vi "Launch App.vi"() -> ()   [LabVIEW 2019]
doc: "Developed by Kevin Thompson\nkevin@thompsonengineering.net\n\nCopyright 2018-2020\nThompson Engineering, LLC"
uses:
  Source/Common/DataTypes/TD GetSet ActionSelect--enum.ctl
  Source/Common/Startup/TD LaunchData--cluster.ctl
  Source/Common/Startup/TD LaunchState--enum.ctl
  Source/Common/Startup/GBL System.vi
  Source/Common/ErrorHandler/ErrorHandler.lvclass
panel:
  out "FP Msg":string="Launching AVC 2.0\nPlease Wait . . ."
  in  "MinimizeLauncher":bool
  out "StatusStr.Launcher":string
  in  "AbortSystemStart":bool
  out "AppVer":string="Ichor Systems AVC2 - Development Mode" caption="Version:"
  # "Launching AVC 2.0\nPlease Wait . . ."
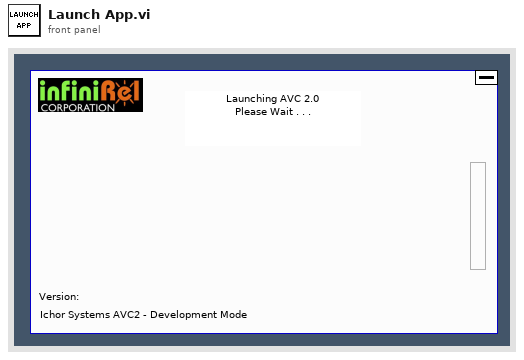
[diagram p1: front panel]
types:
  T1 = typedef "TD GetSet ActionSelect--enum.ctl" = enum16{"Init", "Get", "Set"}
  T2 = enum32{"Invalid", "Default", "Floating", "Floating/Auto-Hide", "Modal"}
  T3 = enum32{"invalid app kind", "Development System", "Run Time System", "Student Edition", "Embedded LabVIEW", "Evaluation", "Custom"}
  T4 = enum32{"Invalid", "Standard", "Closed", "Hidden", "Minimized", "Maximized"}
  T5 = typedef "TD LaunchState--enum.ctl" = enum16{"Started", "Stopped"}
  T6 = typedef "TD LaunchData--cluster.ctl" = cluster{"Time Stamp":timestamp, "LaunchState":T5, "Error":errorcluster}
  T7 = typedef "TD Pathnames--cluster.ctl" = cluster{"RunTimeSys?":bool, "AppFolder":path, "ExecutablePath":path, "ConfigFolder":path, "DataLogFolder":path, "SystemLogFolder":path, "SeqFolder":path, "MainStartupPathname":path, "MainUIPathname":path, "SystemEventsFile":path, "SeqEventsFile":path, "Config SettingsFile":path, "DAQ IOConfigFile":path, "SystemSimulation":bool}
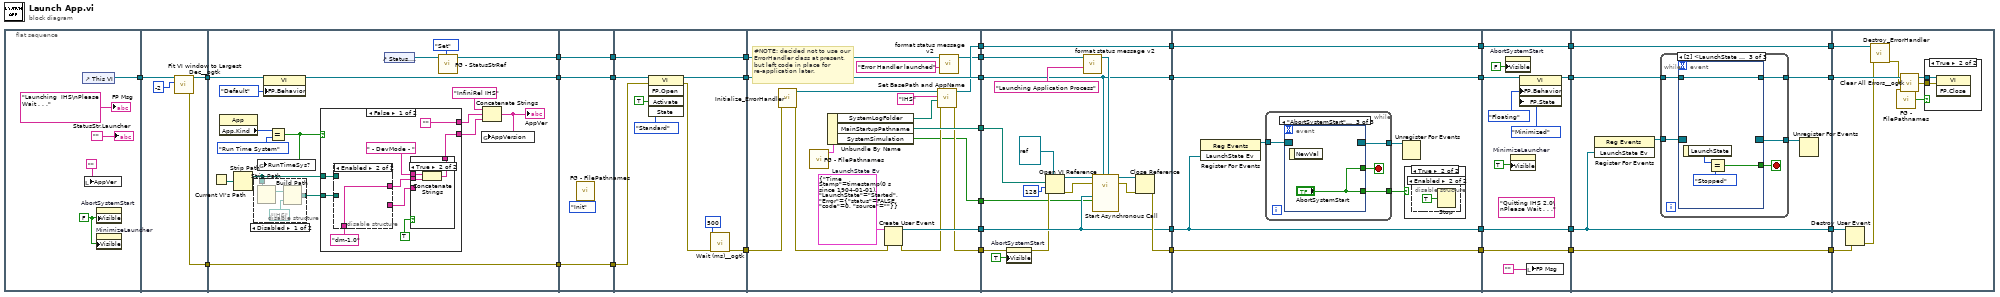
[diagram p0: block diagram]
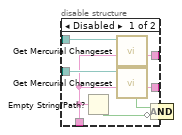
[diagram p3: hidden frame]
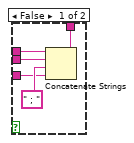
[diagram p4: hidden frame]
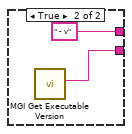
[diagram p5: hidden frame]
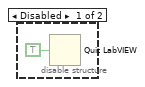
[diagram p7: hidden frame]
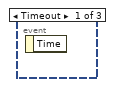
[diagram p8: hidden frame]
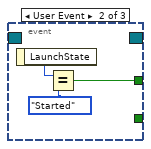
[diagram p9: hidden frame]
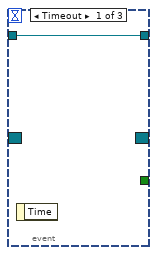
[diagram p10: hidden frame]
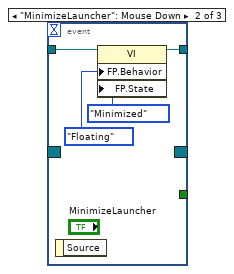
[diagram p11: hidden frame]
diagram:
  n1 = flat-sequence {
    tunnel: [w40] -> w12
    tunnel: [w42] -> w35
    tunnel: [w41] -> w34
    tunnel: w12 -> [w43]
    tunnel: w35 -> [w53]
    tunnel: w34 -> [w56]
    tunnel: [w56] -> w32
    tunnel: [w52] -> w30
    tunnel: [w48] -> w1
    tunnel: w32 -> [w96]
    tunnel: [w96] -> w31
    tunnel: w30 -> [w95]
    tunnel: [w95] -> w29
    tunnel: [w94] -> w3
    tunnel: w1 -> [w94]
    tunnel: w31 -> [w102]
    tunnel: w29 -> [w103]
    tunnel: [w99] -> w33
    tunnel: [w101] -> w25
    tunnel: w3 -> [w97]
    tunnel: [w97] -> w2
    tunnel: w33 -> [w119]
    tunnel: [w112] -> w28
    tunnel: [w122] -> w27
    tunnel: [w121] -> w26
    tunnel: w25 -> [w121]
    tunnel: [w114] -> w11
    tunnel: [w110] -> w9
    tunnel: [w109] -> w5
    tunnel: [w108] -> w4
    tunnel: w2 -> [w107]
    tunnel: w28 -> [w132]
    tunnel: w27 -> [w134]
    tunnel: w26 -> [w124]
    tunnel: [w135] -> w24
    tunnel: [w134] -> w23
    tunnel: [w124] -> w19
    tunnel: w11 -> [w130]
    tunnel: [w129] -> w10
    tunnel: w9 -> [w129]
    tunnel: w5 -> [w128]
    tunnel: w4 -> [w127]
    tunnel: w24 -> [w147]
    tunnel: w23 -> [w144]
    tunnel: [w147] -> w22
    tunnel: [w144] -> w21
    tunnel: [w142] -> w20
    tunnel: w19 -> [w142]
    tunnel: w10 -> [w141]
    tunnel: [w141] -> w7
    tunnel: w22 -> [w167]
    tunnel: w21 -> [w166]
    tunnel: w20 -> [w164]
    tunnel: [w167] -> w18
    tunnel: [w166] -> w17
    tunnel: [w163] -> w16
    tunnel: [w160] -> w8
    tunnel: w7 -> [w160]
    tunnel: w18 -> [w174]
    tunnel: w17 -> [w172]
    tunnel: w16 -> [w169]
    tunnel: [w174] -> w15
    tunnel: [w168] -> w14
    tunnel: [w172] -> w13
    tunnel: w8 -> [w170]
    tunnel: [w170] -> w6
    tunnel: w15 -> [w195]
    tunnel: w14 -> [w194]
    tunnel: w13 -> [w196]
    tunnel: w6 -> [w193]
    frame #0 {
      w38 = FALSE ("Visible")
      n2 = control-ref of="This VI"() -> (w40:refnum<vi>)
      n3 = local write "AppVer"("") -> ()
      n4 = property on="MinimizeLauncher" class="Bool"("Visible"=w38) -> ()  [unwired: 2 in, 2 out]
      n5 = property on="AbortSystemStart" class="Bool"("Visible"=w38) -> ()  [unwired: 2 in, 2 out]
      "StatusStr.Launcher" <- ""
      "FP Msg" <- "Launching  IHS\nPlease Wait . . ." ("FP Msg")
    }
    frame #1 {
      n6 = call <userlib>:"Fit VI window to Largest Dec__ogtk.vi"("border spacing (2 px)"=-2, "VI Ref (calling VI)"=w43) -> ("error out"=w41:errorcluster, "dup VI Ref"=w42:refnum<vi>)  [unwired: 4 in]
    }
    frame #2 {
      n7 = Current VI's Path() -> (path=w47:path)
      n8 = property class="App"() -> ("App.Kind"=w61:T3)  [unwired: 2 in, 2 out]
      n9 = Strip Path(path=w47) -> (stripped path=w46:path)  [unwired: 1 out]
      n10 = disable-structure shown="Disabled" {
        disable-tunnel: w46 -> [w65 _]
        disable-tunnel: [w62 _] -> w45
        frame Disabled {
          n11 = Strip Path(path=w65) -> (stripped path=w64:path)  [unwired: 1 out]
          n12 = Build Path(base path=w64, name or relative path=path "IHS") -> (appended path=w62:path)
        }
        frame Enabled {
        }
      }
      n13 = property class="VI"(reference=w53, "FP.Behavior"=T2."Default" ("Front Panel Window:Behavior")) -> (reference out=w52:refnum<vi>)  [unwired: 1 in, 1 out]
      n14 = Equal?(x=w61, y=T3."Run Time System" ("Application:Kind")) -> (x = y?=w57:bool)
      n15 = global write "GBL System.vi" "RunTimeSys?"(w57) -> ()
      n16 = case shown="False" w57 {
        tunnel: [w70 w92] -> w59
        tunnel: ["" " - v" ("string")] -> w60
        tunnel: w46 -> [w73 _]
        tunnel: w45 -> [w69 _]
        frame False {
          n17 = disable-structure shown="Enabled" {
            disable-tunnel: w73 -> [w81 _]
            disable-tunnel: [w80 w82] -> w71
            disable-tunnel: w69 -> [w79 _]
            disable-tunnel: [w75 _] -> w68
            disable-tunnel: "dm-1.0" -> [w76 w82]
            frame Disabled {
              n18 = Empty String/Path?(string/path=w76) -> (empty?=w77:bool)
              n19 = call "Get Mercurial Changeset.vi"("not found string (\"\")"=w76, "Path"=w81) -> ("Change Set String"=w80:string)  [unwired: 6 in, 3 out]
              n20 = call "Get Mercurial Changeset.vi"("not found string (\"\")"=w76, "Path"=w79) -> ("Change Set String"=w75:string, "repo error?"=w78:bool)  [unwired: 6 in, 2 out]
              n21 = Compound Arithmetic op=AND(w78, invert w77) -> ()  [unwired: 1 out]
            }
            frame Enabled {
            }
          }
          n22 = case shown="True" TRUE {
            tunnel: " - DevMode - " -> [w87 w90]
            tunnel: w71 -> [w86 w88]
            tunnel: [w85 w89] -> w70
            tunnel: w68 -> [w83 _]
            frame False {
              n23 = Concatenate Strings(w87, w86, " ; ", w83) -> (w85:string)
            }
            frame True {
              n24 = Concatenate Strings(w90, w88) -> (w89:string)
            }
          }
        }
        frame True {
          n25 = call <userlib>:"MGI Get Executable Version.vi"() -> ("Version"=w92:string)  [unwired: 7 in]
        }
      }
      n26 = control-ref of="Status.Launcher"() -> (w50:refnum<vi>)
      n27 = call "FG - StatusStrRef.vi"("StatusStr Ref in"=w50, "action (Get)"=TD_GetSet_ActionSelect--enum."Set") -> ("StatusStr Ref out"=w48:refnum<vi>)  [unwired: 7 in, 1 out]
      n28 = Concatenate Strings("InfiniRel IHS" ("string"), w60, w59) -> (w55:string)
      "AppVer" <- w55
      n29 = global write "GBL System.vi" "AppVersion"(w55) -> ()
    }
    frame #3 {
      n30 = call "FG - FilePathnames.vi"("action (Get)"=TD_GetSet_ActionSelect--enum."Init") -> ()  [unwired: 3 in, 2 out]
    }
    frame #4 {
      n31 = invoke class="VI" method="FP.Open"(reference=w103, error in=w102, "Activate"=TRUE ("Activate?"), "State"=T4."Standard") -> (reference out=w101:refnum<vi>, error out=w100:errorcluster)  [unwired: 1 in, 3 out]
      n32 = call <userlib>:"Wait (ms)__ogtk.vi"("error in (no error)"=w100, "milliseconds to wait"=u32 500) -> ("error out"=w99:errorcluster)  [unwired: 8 in, 1 out]
    }
    frame #5 {
      w120 = T6 {"Time Stamp"=timestamp(0 s since 1904-01-01), "LaunchState"=enum."Started", "Error"={"status"=FALSE, "code"=0, "source"=""}}  # LaunchState Ev
      # "#NOTE: decided not to use our\nErrorHandler class at present,\nbut left code in place for\nre-application later."
      n33 = call "Initialize_ErrorHandler.vi"("error in (no error)"=w119) -> ("error out"=w118:errorcluster, "ErrorHandler out"=w117:refnum<class "ErrorHandler.lvclass">)  [unwired: 9 in]
      n34 = call "FG - FilePathnames.vi"() -> ("FilePaths out"=w116:T7)  [unwired: 4 in, 1 out]
      n35 = Unbundle By Name(w116) -> ("SystemLogFolder"=w115:path, "MainStartupPathname"=w114:path, "SystemSimulation"=w109:bool)
      n36 = Create User Event(user event datatype=w120, error in=w118) -> (user event=w122:refnum<user-event>, error out=w113:errorcluster)
      n37 = call "Set BasePath and AppName.vi"("error in (no error)"=w113, "ErrorLogBasePath"=w115, "AppName"="IHS", "ErrorHandler in"=w117) -> ("error out"=w112:errorcluster, "ErrorHandler out"=w110:refnum<class "ErrorHandler.lvclass">)  [unwired: 6 in]
      n38 = call <vilib>:"format status message v2.vi"("status msg"="Error Handler launched", "Str Refnum"=w107) -> ("Str Refnum out"=w108:refnum<vi>)  [unwired: 5 in, 4 out]
    }
    frame #6 {
      n39 = property on="AbortSystemStart" class="Bool"(error in=w132, "Visible"=TRUE) -> (error out=w131:errorcluster)  [unwired: 1 in, 1 out]
      n40 = Open VI Reference(type specifier VI Refnum (for type only)=refnum<vi> refnum, vi path=w130, options=128, error in (no error)=w131) -> (vi reference=w139:refnum<vi>, error out=w136:errorcluster)  [unwired: 2 in]
      n41 = call <vilib>:"format status message v2.vi"("status msg"="Launching Application Process", "Str Refnum"=w127) -> ("Str Refnum out"=w125:refnum<vi>)  [unwired: 5 in, 4 out]
      n42 = call-by-ref "Start Asynchronous Call"(reference=w139, error in=w136, "Splash StatusRef"=w125, "Splash VI Ref"=w124, "Simulation?"=w128, "LaunchState Ev"=w134) -> (reference out=w138:refnum<vi>, error out=w137:errorcluster)  [unwired: 8 in]
      n43 = Close Reference(reference=w138, error in (no error)=w137) -> (error out=w135:errorcluster)
    }
    frame #7 {
      n44 = register-events(w144) -> (reference out=w146:refnum<event-registration>)  [unwired: 2 in, 1 out]
      n45 = while {
        tunnel: w146 -> [w153]
        tunnel: [w152] -> w145
        tunnel: [w150] -> w143
        stop <- w151 stop-if-true
        n46 = event shown="[2] \"AbortSystemStart\": Value Change" {
          selector: w153 -> [_ _ _]
          dyn-events: [_ _ _] -> w152
          timeout: _ -> [_ _ _]
          tunnel: [_ w154 "AbortSystemStart"] -> w151
          tunnel: [_ _ "AbortSystemStart"] -> w150
          event Timeout {
            n47 = event-data() -> ()  [unwired: 1 in, 1 out]
          }
          event User Event {
            n48 = event-data() -> ("LaunchState"=w156:T5)  [unwired: 1 in]
            n49 = Equal?(x=w156, y=TD_LaunchState--enum."Started") -> (x = y?=w154:bool)
          }
          event "AbortSystemStart": Value Change {
            n50 = event-data() -> ()  [unwired: 1 in, 1 out]
          }
        }
      }
      n51 = Unregister For Events(event registration refnum=w145) -> ()  [unwired: 1 in, 1 out]
      n52 = case shown="True" w143 {
        frame False {
        }
        frame True {
          n53 = disable-structure shown="Enabled" {
            frame Disabled {
              n54 = Quit LabVIEW(quit? (T)=TRUE) -> ()
            }
            frame Enabled {
              n55 = Stop(stop? (T)=TRUE) -> ()
            }
          }
        }
      }
    }
    frame #8 {
      (unwired) "Quitting IHS 2.0\nPlease Wait . . ." ("FP Msg")
      n56 = property on="AbortSystemStart" class="Bool"("Visible"=FALSE) -> ()  [unwired: 2 in, 2 out]
      n57 = property on="MinimizeLauncher" class="Bool"("Visible"=TRUE) -> ()  [unwired: 2 in, 2 out]
      n58 = property class="VI"(reference=w164, "FP.Behavior"=T2."Floating" ("Front Panel Window:Behavior"), "FP.State"=T4."Minimized" ("Front Panel Window:State")) -> (reference out=w163:refnum<vi>)  [unwired: 1 in, 1 out]
      n59 = local write "FP Msg"("") -> ()
    }
    frame #9 {
      n60 = register-events(w172) -> (reference out=w173:refnum<event-registration>)  [unwired: 2 in, 1 out]
      n61 = while {
        tunnel: w173 -> [w179]
        tunnel: [w178] -> w171
        tunnel: w169 -> [w176]
        tunnel: [w175] -> w168
        stop <- w177 stop-if-true
        n62 = event shown="[2] <LaunchState Ev>: User Event" {
          selector: w179 -> [_ _ _]
          dyn-events: [_ _ _] -> w178
          timeout: _ -> [_ _ _]
          tunnel: [_ _ w186] -> w177
          tunnel: w176 -> [w180 w182 w185]
          tunnel: [w180 w181 w185] -> w175
          event Timeout {
            n63 = event-data() -> ()  [unwired: 1 in, 1 out]
          }
          event "MinimizeLauncher": Mouse Down {
            n64 = event-data() -> ()  [unwired: 1 in, 1 out]
            n65 = property class="VI"(reference=w182, "FP.Behavior"=T2."Floating" ("Front Panel Window:Behavior"), "FP.State"=T4."Minimized" ("Front Panel Window:State")) -> (reference out=w181:refnum<vi>)  [unwired: 1 in, 1 out]
          }
          event User Event {
            n66 = event-data() -> ("LaunchState"=w188:T5)  [unwired: 1 in]
            n67 = Equal?(x=w188, y=TD_LaunchState--enum."Stopped") -> (x = y?=w186:bool)
          }
        }
      }
      n68 = Unregister For Events(event registration refnum=w171) -> ()  [unwired: 1 in, 1 out]
    }
    frame #10 {
      n69 = Destroy User Event(user event=w196, error in=w195) -> (error out=w191:errorcluster)
      n70 = call "Destroy_ErrorHandler.vi"("error in (no error)"=w191, "ErrorHandler in"=w193) -> ("error out"=w192:errorcluster)  [unwired: 8 in, 1 out]
      n71 = call "FG - FilePathnames.vi"() -> ("RunTimeSys?"=w189:bool)  [unwired: 4 in, 1 out]
      n72 = call <userlib>:"Clear All Errors__ogtk.vi"("Error In"=w192) -> ("Error Out"=w190:errorcluster)  [unwired: 3 in]
      n73 = case shown="True" w189 {
        tunnel: w194 -> [_ w198]
        tunnel: w190 -> [_ w197]
        frame False {
        }
        frame True {
          n74 = invoke class="VI" method="FP.Close"(reference=w198, error in=w197) -> ()  [unwired: 1 in, 3 out]
        }
      }
    }
  }
